vi "Write Update UI Event.vi"(10 "Update UI Event":refnum<user-event>, 11 "Timing Engine in":refnum<class "Timing Engine.lvclass">) -> (3 "Timing Engine out":refnum<class "Timing Engine.lvclass">)   [LabVIEW 2016, in "Assert Display.lvlib" / "Timing Engine.lvlib" / "Timing Engine.lvclass"]
uses:
  Timing Engine.lvclass
  Timing Engine.lvclass/Timing Engine.ctl
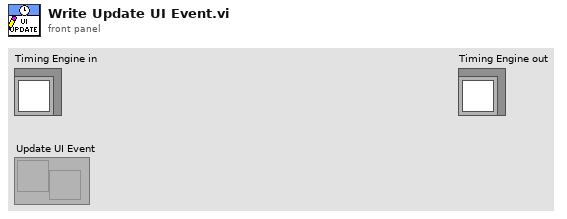
[diagram p1: front panel]
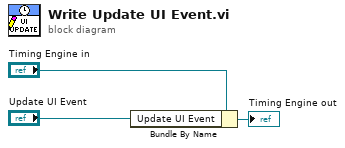
[diagram p0: block diagram]
diagram:
  n1 = Bundle By Name(cluster="Timing Engine in", "Update UI Event"="Update UI Event") -> (→"Timing Engine out":refnum<class "Timing Engine.lvclass">)
